vi "Get Power Meter Result.vi"(0 "SG Path in":refnum<class "SG Abstract Path.lvclass">, 5 "Cal point in":T1, 11 "error in (no error)":errorcluster) -> (4 "SG Path out":refnum<class "SG Abstract Path.lvclass">, 8 "Power (dBm)":dbl, 15 "error out":errorcluster)   [LabVIEW 2023, in "RFFixtureCharact.Public.lvlib" / "SG Abstract Path.lvclass"]
uses:
  SG Abstract Path.lvclass
  Scalar Path/Type Definitions/Cal Point.ctl
  SG Abstract Path.lvclass/SG Abstract Path.ctl
  Instruments/Power Meter/SG Path PM Accessor Base/SG Path PM Accessor Base.lvclass
  Scalar Path/Scalar Path.lvclass
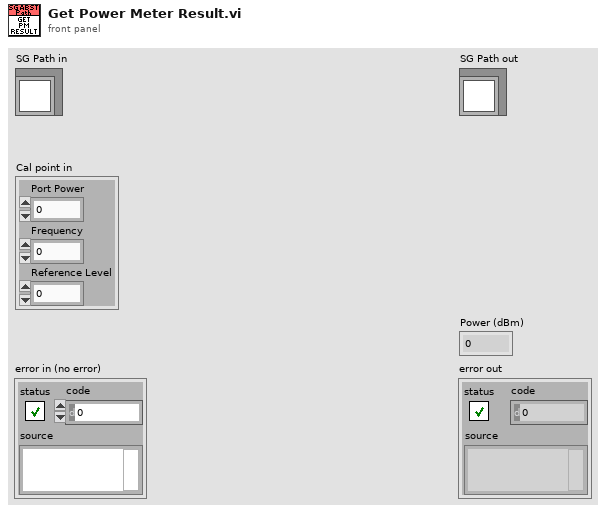
[diagram p1: front panel]
types:
  T1 = typedef "RFFixtureCharact.Public.lvlib/Scalar Path.lvclass/Cal Point.ctl" = cluster{"Port Power":dbl, "Frequency":dbl, "Reference Level":dbl}
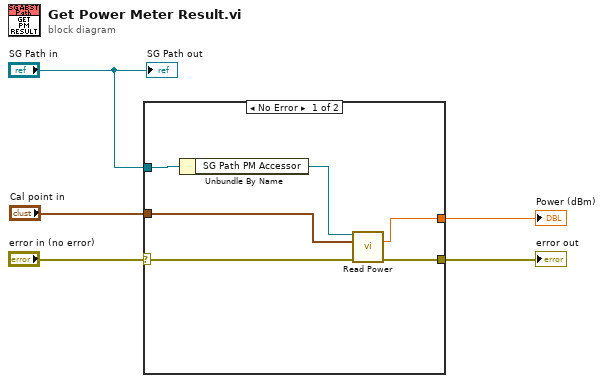
[diagram p0: block diagram]
diagram:
  n1 = case shown="No Error" "error in (no error)" {
    selector: "error in (no error)" -> [w10 w12]
    tunnel: [w9 w12] -> w4
    tunnel: "SG Path in" -> [w11 _]
    tunnel: [w7 _] -> w2
    tunnel: "Cal point in" -> [w6 _]
    frame No Error {
      n2 = Unbundle By Name(w11) -> ("SG Path PM Accessor"=w8:refnum<class "SG Path PM Accessor Base.lvclass">)
      n3 = call-dynamic "Read Power.vi"("SG Path Power Meter Accessor in"=w8, "Cal point in"=w6, "error in (no error)"=w10) -> ("Power (dBm)"=w7:dbl, "error out"=w9:errorcluster)  [unwired: 10 in, 1 out]
    }
    frame Error {
    }
  }
  "error out" <- w4
  "Power (dBm)" <- w2
  "SG Path out" <- "SG Path in"
